vi "Build Edge Context Menu.vi"(0 "Display State In":T1, 5 "Edges":refnum<class "FSM.Edge.lvclass">[](array[class]), 7 "Names":string[](array[string]), 9 "Tags":string[](array[string]), 11 "menu ref":refnum<k9>) -> ()   [LabVIEW 2015, in "FSM Editor.xctl"]
uses:
  FSM Editor.xctl
  State.vi
  Classes/FSM.Port/FSM.Port.lvclass
  <vilib>/Utility/miscctls.llb/LVPoint32TypeDef.ctl
  Drag Mode.ctl
  Events.ctl
  NodeAdded.ctl
  NodeSelected.ctl
  EdgeEventData.ctl
  Classes/FSM.Edge/FSM.Edge.lvclass
  Classes/FSM.Edge/FSM.Edge.lvclass/FSM.Edge.ctl
  Classes/FSM.Label/FSM.Label.lvclass/FSM.Label.ctl
  Classes/FSM.Edge/Read Type.vi
  Classes/FSM.Edge/Read Label.vi
  Classes/FSM.Label/Read Text.vi
  Classes/FSM.Label/FSM.Label.lvclass
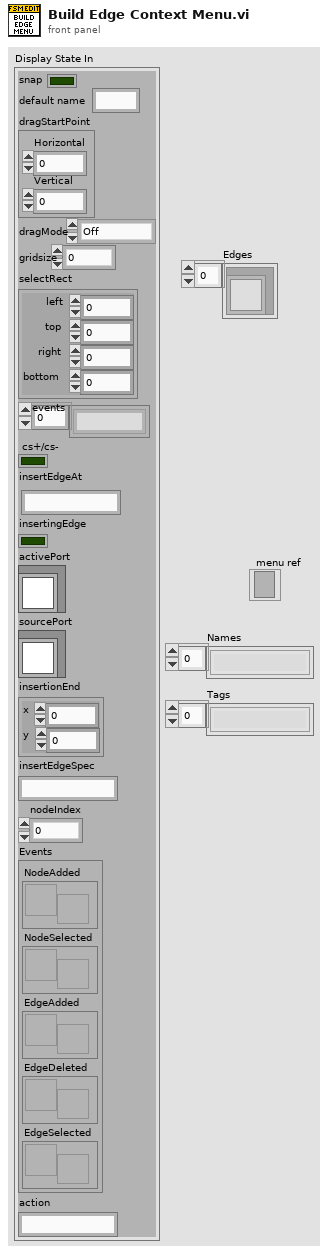
[diagram p1: front panel]
types:
  T1 = typedef "FSM Editor.xctl/State.vi" = cluster{"snap":bool, "default name":string, "dragStartPoint":T2, "dragMode":T3, "gridsize":dbl, "selectRect":cluster{"left":i16, "top":i16, "right":i16, "bottom":i16}, "events":string[], "cs+/cs-":bool, "insertEdgeAt":string, "insertingEdge":bool, "activePort":refnum<class "FSM.Port.lvclass">, "sourcePort":refnum<class "FSM.Port.lvclass">, "insertionEnd":cluster{"x":i16, "y":i16}, "insertEdgeSpec":string, "nodeIndex":i32, "Events":T4, "action":string}
  T2 = typedef "LVPoint32TypeDef.ctl" = cluster{"Horizontal":i32, "Vertical":i32}
  T3 = typedef "Drag Mode.ctl" = enum16{"Off", "NodePending", "Nodes", "Pan", "Select", "EdgeInsertion", "EdgePoint", "EdgeLabel"}
  T4 = typedef "FSM Editor.xctl/Events.ctl" = cluster{"NodeAdded":refnum<user-event>, "NodeSelected":refnum<user-event>, "EdgeAdded":refnum<user-event>, "EdgeDeleted":refnum<user-event>, "EdgeSelected":refnum<user-event>}
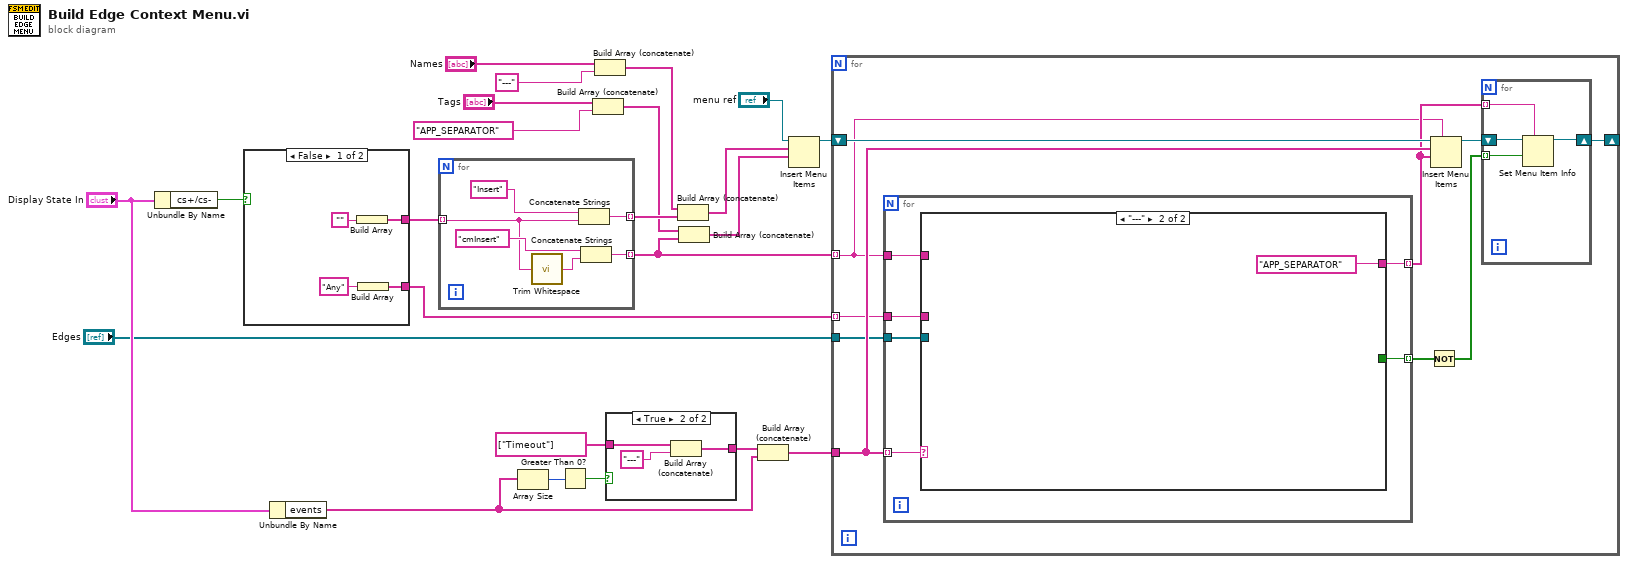
[diagram p0: block diagram]
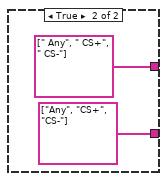
[diagram p3: hidden frame]
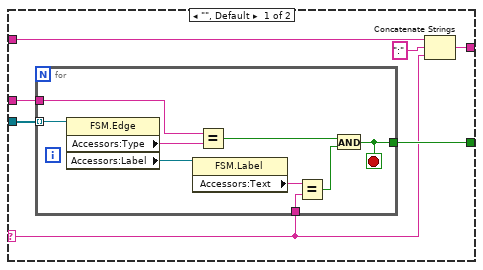
[diagram p4: hidden frame]
diagram:
  n1 = Unbundle By Name("Display State In") -> ("cs+/cs-"=w19:bool)
  n2 = case shown="False" w19 {
    tunnel: [w27 string[] [" Any", " CS+", " CS-"]] -> w3
    tunnel: [w25 string[] ["Any", "CS+", "CS-"]] -> w1
    frame False {
      n3 = Build Array("") -> (w27:string[])
      n4 = Build Array("Any") -> (w25:string[])
    }
    frame True {
    }
  }
  n5 = Unbundle By Name("Display State In") -> ("events"=w6:string[])
  n6 = for {
    tunnel: w3 -> [w33] mode=indexing
    tunnel: [w32] -> w17 mode=indexing
    tunnel: [w31] -> w4 mode=indexing
    n7 = call <vilib>:"Trim Whitespace.vi"("string"=w33) -> ("trimmed string"=w30:string)  [unwired: 1 in]
    n8 = Concatenate Strings("Insert", w33) -> (w32:string)
    n9 = Concatenate Strings("cmInsert", w30) -> (w31:string)
  }
  n10 = Array Size(array=w6) -> (size(s)=w10:i32)
  n11 = Greater Than 0?(x=w10) -> (x > 0?=w9:bool)
  n12 = Build Array (concatenate)("Tags", "APP_SEPARATOR") -> (w15:string[])
  n13 = Build Array (concatenate)("Names", "---") -> (w16:string[])
  n14 = case shown="True" w9 {
    tunnel: string[] ["Timeout"] -> [w36 w39]
    tunnel: [w36 w37] -> w7
    frame False {
    }
    frame True {
      n15 = Build Array (concatenate)(w39, "---") -> (w37:string[])
    }
  }
  n16 = Build Array (concatenate)(w16, w17) -> (w13:string[])
  n17 = Build Array (concatenate)(w15, w4) -> (w11:string[])
  n18 = Build Array (concatenate)(w7, w6) -> (w5:string[])
  n19 = Insert Menu Items(7:w11, 8:w13, 9:"menu ref") -> (3:w12:refnum<k9>)  [unwired: 3 in, 2 out]
  n20 = for {
    shift-right: [w45] -> _
    shift-left: w12 -> [w49]
    tunnel: w4 -> [w40] mode=indexing
    tunnel: w5 -> [w48]
    tunnel: w1 -> [w42] mode=indexing
    tunnel: "Edges" -> [w47]
    n21 = for {
      tunnel: w48 -> [w55] mode=indexing
      tunnel: [w54] -> w44 mode=indexing
      tunnel: w47 -> [w53]
      tunnel: [w52] -> w43 mode=indexing
      tunnel: w42 -> [w51]
      tunnel: w40 -> [w50]
      n22 = case shown="\"---\"" w55 {
        selector: w55 -> [w57 _]
        tunnel: [w58 "APP_SEPARATOR"] -> w54
        tunnel: w53 -> [w62 _]
        tunnel: [w61 _] -> w52
        tunnel: w51 -> [w60 _]
        tunnel: w50 -> [w59 _]
        frame "", Default {
          n23 = for {
            tunnel: w62 -> [w71] mode=indexing
            tunnel: [w63] -> w61
            tunnel: w57 -> [w69]
            tunnel: w60 -> [w64]
            stop <- w63 stop-if-true
            n24 = property class="FSM.Edge"(reference=w71) -> ("Accessors:Type"=w66:string, "Accessors:Label"=w67:refnum<class "FSM.Label.lvclass">)  [unwired: 1 in, 2 out]
            n25 = property class="FSM.Label"(reference=w67) -> ("Accessors:Text"=w70:string)  [unwired: 1 in, 2 out]
            n26 = Equal?(x=w64, y=w66) -> (x = y?=w65:bool)
            n27 = Equal?(x=w70, y=w69) -> (x = y?=w68:bool)
            n28 = And(x=w65, y=w68) -> (x .and. y?=w63:bool)
          }
          n29 = Concatenate Strings(w59, ":" ("string"), w57) -> (w58:string)
        }
        frame "---" {
        }
      }
    }
    n30 = Not(x=w43) -> (.not. x?=w41:bool[])
    n31 = Insert Menu Items(5:w40, 7:w44, 8:w48, 9:w49) -> (3:w46:refnum<k9>)  [unwired: 2 in, 2 out]
    n32 = for {
      shift-right: [w75] -> w45
      shift-left: w46 -> [w76]
      tunnel: w44 -> [w74] mode=indexing
      tunnel: w41 -> [w73] mode=indexing
      n33 = Set Menu Item Info(7:w74, 9:w73, 11:w76) -> (3:w75:refnum<k9>)  [unwired: 4 in, 1 out]
    }
  }
